vi "Handler - Data Timeout.vi"(8 "error in (no error)":errorcluster, 10 "Timeout Array":bool[](array[boolean]), 11 "Data Timestamp":timestamp) -> (0 "error out":errorcluster)   [LabVIEW 2018]
doc: "If there was a timeout among the shared variables even though the first variable did not timeout, something is wrong and data may be missing. Send a strong to the log file on the Host."
uses:
  RT - Host Comms/RT - Host Comms.lvlib
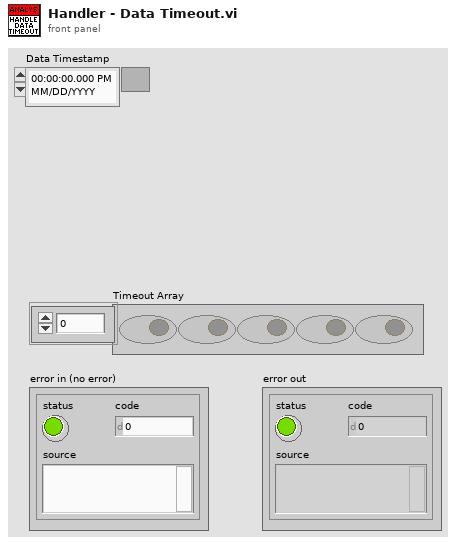
[diagram p1: front panel]
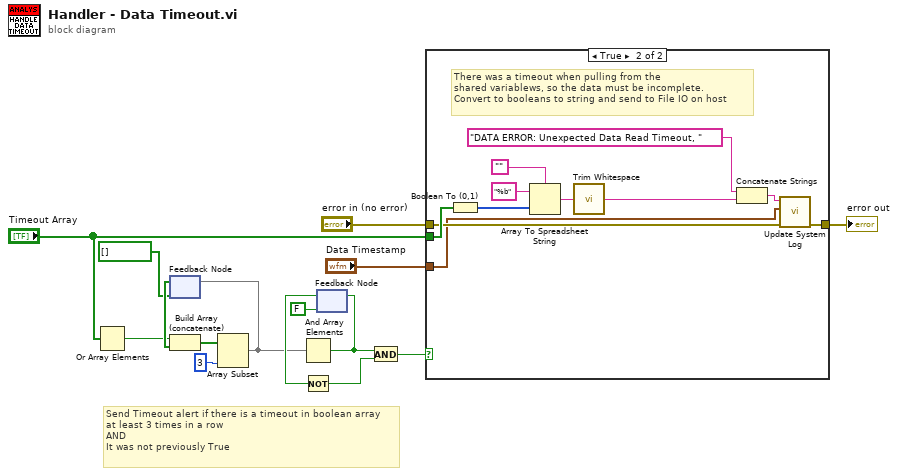
[diagram p0: block diagram]
diagram:
  # "Send Timeout alert if there is a timeout in boolean array\nat least 3 times in a row\nAND\nIt was not previously True"
  n1 = Or Array Elements(Boolean array="Timeout Array") -> (logical OR=w2:bool)
  n2 = feedback #1(bool[] []) -> (w11:bool[])
  n3 = Build Array (concatenate)(w2, w11) -> (w8:bool[])
  n4 = Array Subset(array=w8, length=3) -> (w1:bool[])  [unwired: 1 in]
  n5 = feedback-in #1(w1) -> ()
  n6 = And Array Elements(Boolean array=w1) -> (logical AND=w3:bool)
  n7 = feedback #2(FALSE) -> (w6:bool)
  n8 = Not(x=w6) -> (.not. x?=w4:bool)
  n9 = feedback-in #2(w3) -> ()
  n10 = And(x=w3, y=w4) -> (x .and. y?=w7:bool)
  n11 = case shown="True" w7 {
    tunnel: "Data Timestamp" -> [_ w17]
    tunnel: [w16 w19] -> w13
    tunnel: "error in (no error)" -> [w16 w20]
    tunnel: "Timeout Array" -> [_ w27]
    frame False {
    }
    frame True {
      # "There was a timeout when pulling from the \nshared variablews, so the data must be incomplete.\nConvert to booleans to string and send to File IO on host"
      n12 = Boolean To (0,1)(Boolean=w27) -> (0, 1=w22:i16[])
      n13 = Array To Spreadsheet String(delimiter (Tab)="", array=w22, 3:"%b" ("format string")) -> (spreadsheet string=w25:string)
      n14 = call <vilib>:"Trim Whitespace.vi"("string"=w25) -> ("trimmed string"=w24:string)  [unwired: 1 in]
      n15 = Concatenate Strings("DATA ERROR: Unexpected Data Read Timeout, " ("string"), w24) -> (w18:string)
      n16 = call "Update System Log.vi"("error in (no error)"=w20, "time stamp"=w17, "Message"=w18) -> ("error out"=w19:errorcluster)  [unwired: 8 in]
    }
  }
  "error out" <- w13
